vi "Test Camera.vi"() -> ()   [LabVIEW 2021]
uses:
  Camera/Camera.lvclass
  Canon/Canon.lvclass
  C:/Projects/InstrPanel/Classes/Camera/Camera.lvclass
  Nikon/Nikon.lvclass
panel:
  in  "Nikon Data":string="NikonCustom"
  in  "Canon Data":string="CanonCustom"
  out "Data":string[](array[string])
  in  "Status":bool=TRUE
  in  "Cycles":i32=14
  in  "Name":string="ThisisLuis"
  in  "Type":enum16{"Camera", "Canon", "Nikon"}(ring)
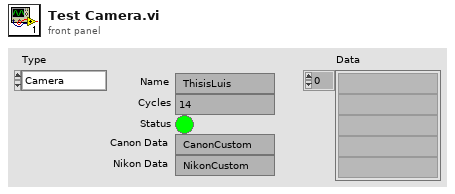
[diagram p1: front panel]
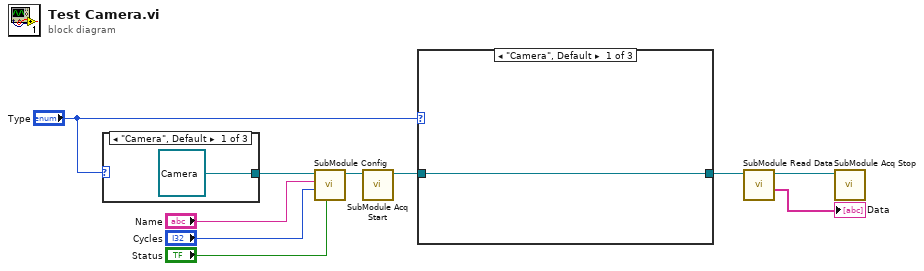
[diagram p0: block diagram]
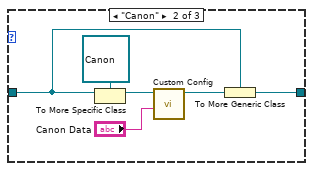
[diagram p2: hidden frame]
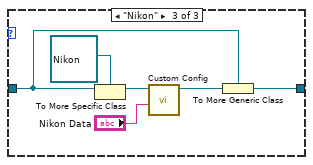
[diagram p3: hidden frame]
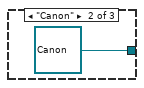
[diagram p4: hidden frame]
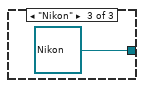
[diagram p5: hidden frame]
diagram:
  n1 = case shown="\"Camera\", Default" "Type" {
    tunnel: [refnum<class "Camera.lvclass"> refnum ("Camera.lvclass") refnum<class "Canon.lvclass"> refnum ("Canon.lvclass") refnum<class "Nikon.lvclass"> refnum ("Nikon.lvclass")] -> w10
    frame "Camera", Default {
    }
    frame "Canon" {
    }
    frame "Nikon" {
    }
  }
  n2 = call-dynamic "SubModule Config.vi"("Status"="Status", "Cycles"="Cycles", "Name"="Name", "Camera in"=w10) -> ("Camera out"=w9:refnum<class "Camera.lvclass">)  [unwired: 6 in, 1 out]
  n3 = call-dynamic "SubModule Acq Start.vi"("Camera in"=w9) -> ("Camera out"=w3:refnum<class "Camera.lvclass">)  [unwired: 9 in, 1 out]
  n4 = case shown="\"Camera\", Default" "Type" {
    tunnel: [w14 w16 w22] -> w4
    tunnel: w3 -> [w14 w15 w21]
    frame "Camera", Default {
    }
    frame "Canon" {
      n5 = To More Specific Class(target class=refnum<class "Canon.lvclass"> refnum ("Canon.lvclass"), reference=w15) -> (specific class reference=w19:refnum<class "Canon.lvclass">)  [unwired: 1 in, 1 out]
      n6 = call "Custom Config.vi"("Canon Data"="Canon Data", "Canon in"=w19) -> ("Canon out"=w20:refnum<class "Canon.lvclass">)  [unwired: 8 in, 1 out]
      n7 = To More Generic Class(target class=w15, reference=w20) -> (generic class reference=w16:refnum<class "Camera.lvclass">)
    }
    frame "Nikon" {
      n8 = To More Specific Class(target class=refnum<class "Nikon.lvclass"> refnum ("Nikon"), reference=w21) -> (specific class reference=w25:refnum<class "Nikon.lvclass">)  [unwired: 1 in, 1 out]
      n9 = call "Custom Config.vi"("Nikon Data"="Nikon Data", "Nikon in"=w25) -> ("Nikon out"=w26:refnum<class "Nikon.lvclass">)  [unwired: 8 in, 1 out]
      n10 = To More Generic Class(target class=w21, reference=w26) -> (generic class reference=w22:refnum<class "Camera.lvclass">)
    }
  }
  n11 = call-dynamic "SubModule Read Data.vi"("Camera in"=w4) -> ("Data"=→"Data":string[], "Camera out"=w8:refnum<class "Camera.lvclass">)  [unwired: 8 in, 1 out]
  n12 = call-dynamic "SubModule Acq Stop.vi"("Camera in"=w8) -> ()  [unwired: 9 in, 2 out]
